vi "Initialise Base Actor.vi"(6 "Name":string, 8 "error in (no error)":errorcluster, 10 "Received Messages Channel":refnum<user-event>, 11 "Actor in":refnum<class "Actor.lvclass">) -> (0 "error out":errorcluster, 3 "Actor out":refnum<class "Actor.lvclass">)   [LabVIEW 2020, in "Actor.lvclass"]
uses:
  Actor.lvclass
  Message.ctl
  Actor.lvclass/Actor.ctl
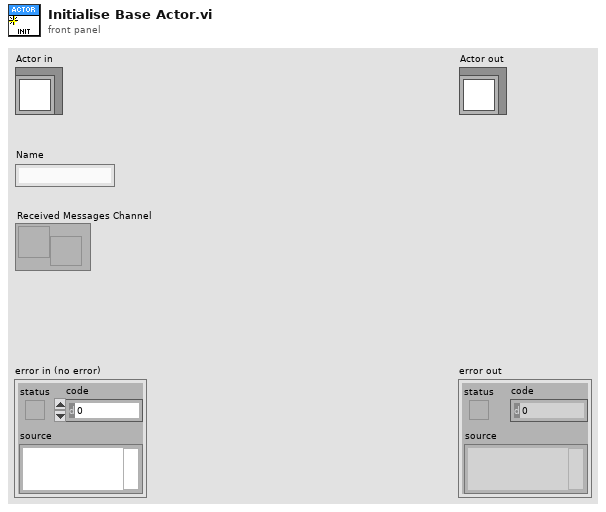
[diagram p1: front panel]
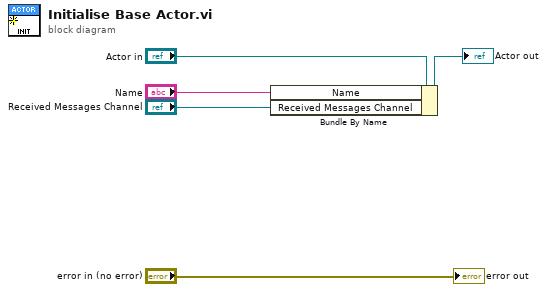
[diagram p0: block diagram]
diagram:
  n1 = Bundle By Name(cluster="Actor in", "Name"="Name", "Received Messages Channel"="Received Messages Channel") -> (→"Actor out":refnum<class "Actor.lvclass">)
  "error out" <- "error in (no error)"
